vi "MGCC_StaEst_main_v3.vi"() -> ()   [LabVIEW 2016]
doc: "This VI is designed for the state estimation function block. The current version is designed for IEEE13node system. The advanced model will be available in the latest version. There is no input for this VI. Bascially, the input right now comes from the cvs in IEEE13 folder."
panel:
  out "index":i32
  out "error out":errorcluster
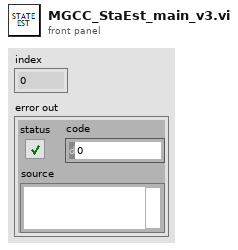
[diagram p1: front panel]
types:
  T1 = cluster{"V_node":cdb[][], "P_node":cdb[][], "I_node":cdb[][], "NumN":dbl, "NumL":dbl, "Ybus":cdb[][], "sspn":dbl[][], "ssqn":dbl[][], "ssvn":dbl[][], "SlackBus":dbl, "Topology":dbl[][]}
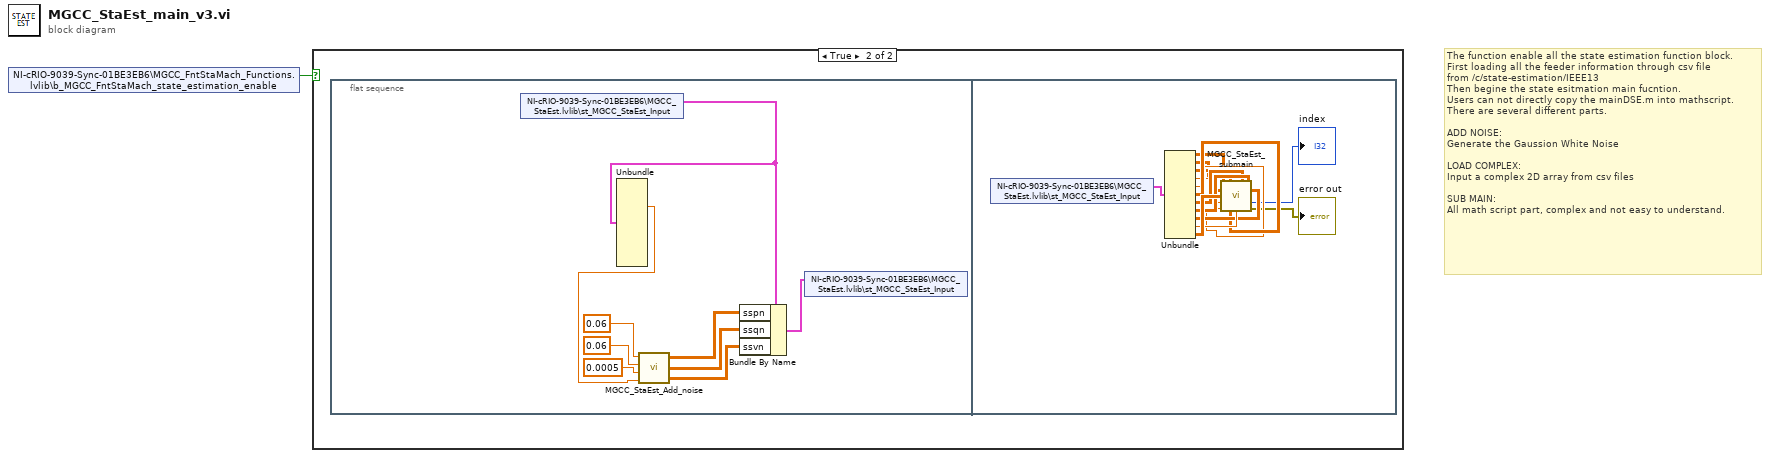
[diagram p0: block diagram]
diagram:
  # "The function enable all the state estimation function block.\nFirst loading all the feeder information through csv file\nfrom /c/state-estimation/IEEE13\nThen begine the state esitmation main fucntion.\nUsers can not directly copy the mainDSE.m into mathscript.\nThere are several different parts.\n\nADD NOISE:\nGenerate the Gaussion White Noise\n\nLOAD COMPLEX:\nInput a complex 2D array from csv files\n\nSUB MAIN:\nAll math script part, complex and not easy to understand."
  n1 = shared-variable "NI-cRIO-9039-Sync-01BE3EB6\\MGCC_FntStaMach_Functions.lvlib\\b_MGCC_FntStaMach_state_estimation_enable"() -> (w1:bool)  [unwired: 1 in, 1 out]
  n2 = case shown="True" w1 {
    frame False {
    }
    frame True {
      n3 = flat-sequence {
        frame #0 {
          n4 = shared-variable "NI-cRIO-9039-Sync-01BE3EB6\\MGCC_StaEst.lvlib\\st_MGCC_StaEst_Input"() -> (w3:T1)  [unwired: 1 in, 1 out]
          n5 = Unbundle(w3) -> ("NumN"=w2:dbl)  [unwired: 10 out]
          n6 = call "MGCC_StaEst_Add_noise.vi"("Node"=w2, "svn"=0.0005, "sqn"=0.06, "spn"=0.06) -> ("ssvn"=w4:dbl[][], "ssqn"=w5:dbl[][], "sspn"=w6:dbl[][])
          n7 = Bundle By Name(cluster=w3, "sspn"=w6, "ssqn"=w5, "ssvn"=w4) -> (w10:T1)
          n8 = shared-variable "NI-cRIO-9039-Sync-01BE3EB6\\MGCC_StaEst.lvlib\\st_MGCC_StaEst_Input"(w10) -> ()  [unwired: 1 in, 1 out]
        }
        frame #1 {
          n9 = shared-variable "NI-cRIO-9039-Sync-01BE3EB6\\MGCC_StaEst.lvlib\\st_MGCC_StaEst_Input"() -> (w24:T1)  [unwired: 1 in, 1 out]
          n10 = Unbundle(w24) -> ("V_node"=w13:cdb[][], "P_node"=w14:cdb[][], "I_node"=w15:cdb[][], "NumN"=w16:dbl, "NumL"=w17:dbl, "Ybus"=w18:cdb[][], "sspn"=w19:dbl[][], "ssqn"=w20:dbl[][], "ssvn"=w21:dbl[][], "SlackBus"=w22:dbl, "Topology"=w23:dbl[][])
          n11 = call "MGCC_StaEst_submain.vi"("V_node"=w13, "I_node"=w15, "sspn"=w19, "ssqn"=w20, "P_node"=w14, "ssvn"=w21, "Topology"=w23, "NumN"=w16, "NumL"=w17, "Ybus"=w18, "SlackBus"=w22) -> ("index"=→"index":i32, "error out"=→"error out":errorcluster)  [unwired: 3 in]
        }
      }
    }
  }
